vi "Read.vi"() -> ()   [LabVIEW 2017]
uses:
  <vilib>/Instr/_visa.llb/VISA Flush IO Buffer Mask.ctl
  <vilib>/Instr/_visa.llb/VISA Configure Serial Port (Instr).vi
panel:
  out "Waveform":i32(graph)
  out "read buffer":string
  in  "Start":bool
  in  "USB Port":refnum<visa-resource-name>
  in  "baud rate (115200)":u32=9600
  in  "parity (0:none)":enum16{"None", "Odd", "Even", "Mark", "Space"}(ring)
  in  "data bits (8)":u16=8 min=5 max=8 step=1
  in  "stop bits (10: 1 bit)":u16(ring)=10 items=["1.0"=10, "1.5"=15, "2.0"=20]
  in  "flow control (0:none)":u16(ring) items=["None", "XON/XOFF", "RTS/CTS", "XON/XOFF & RTS/CTS", "DTR/DSR", "XON/XOFF & DTR/DSR"]
  # "Designed By : Pouya Mansournia"
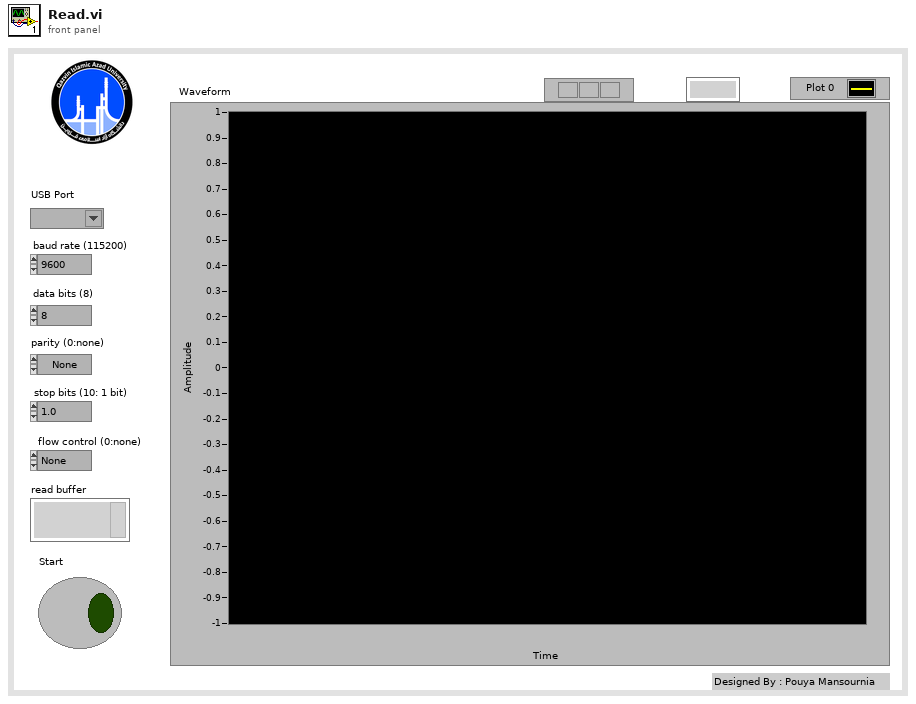
[diagram p1: front panel]
types:
  T1 = typedef "VISA Flush IO Buffer Mask.ctl" = u16
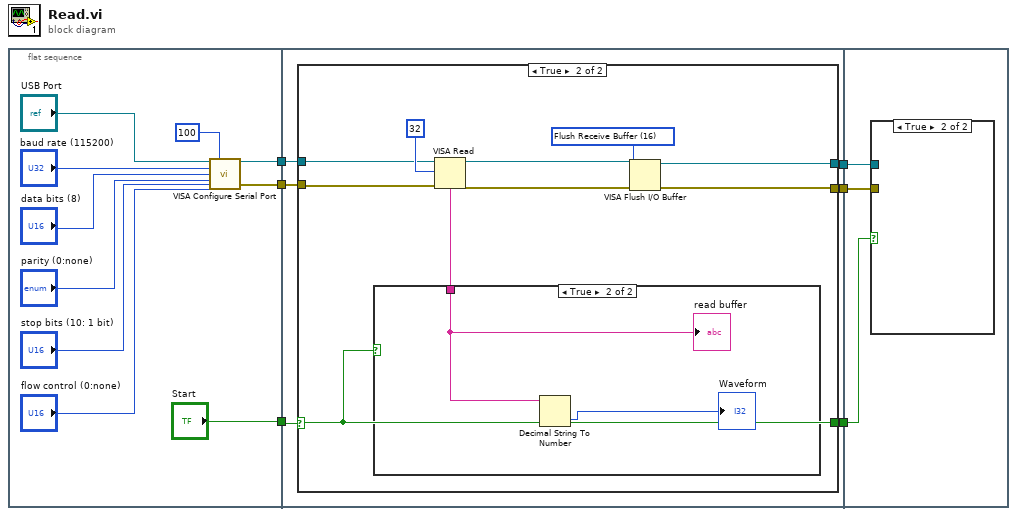
[diagram p0: block diagram]
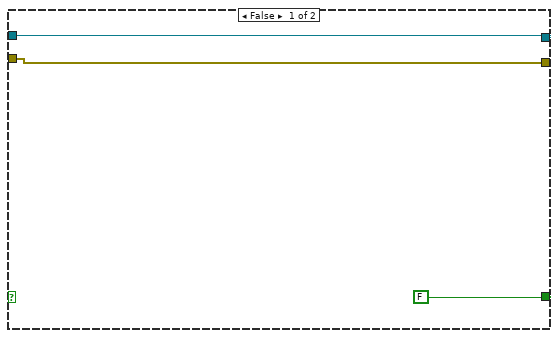
[diagram p2: hidden frame]
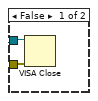
[diagram p4: hidden frame]
diagram:
  n1 = flat-sequence {
    tunnel: [w9] -> w6
    tunnel: [w10] -> w5
    tunnel: ["Start"] -> w2
    tunnel: w6 -> [w22]
    tunnel: w5 -> [w21]
    tunnel: [w20] -> w4
    tunnel: [w19] -> w3
    tunnel: w2 -> [w17]
    tunnel: [w18] -> w1
    tunnel: w4 -> [w40]
    tunnel: w3 -> [w39]
    tunnel: w1 -> [w38]
    frame #0 {
      n2 = call-poly "VISA Configure Serial Port"("VISA resource name"="USB Port", "timeout (10sec)"=u32 100, "baud rate (9600)"="baud rate (115200)", "data bits (8)"="data bits (8)", "parity (0:none)"="parity (0:none)", "stop bits (10: 1 bit)"="stop bits (10: 1 bit)", "flow control (0:none)"="flow control (0:none)") -> ("VISA resource name out"=w9:refnum<visa-resource-name>, "error out"=w10:errorcluster)  [unwired: 7 in]
    }
    frame #1 {
      n3 = case shown="True" w17 {
        selector: w17 -> [_ w29]
        tunnel: w22 -> [w25 w31]
        tunnel: w21 -> [w24 w26]
        tunnel: [w25 w30] -> w20
        tunnel: [w24 w28] -> w19
        tunnel: [FALSE w29] -> w18
        frame False {
        }
        frame True {
          w35 = T1 16 items=["Flush Receive Buffer"=16, "Write Transmit Buffer to Device"=32, "Flush Receive Buffer (No I/O)"=64, "Flush Transmit Buffer"=128] ("Mask")
          n4 = VISA Read(VISA resource name=w31, byte count=u32 32, error in (no error)=w26) -> (VISA resource name out=w34:refnum<visa-resource-name>, read buffer=w32:string, error out=w27:errorcluster)  [unwired: 1 out]
          n5 = case shown="True" w29 {
            tunnel: w32 -> [_ w37]
            frame False {
            }
            frame True {
              n6 = Decimal String To Number(string=w37) -> (number=→"Waveform":i32)  [unwired: 2 in, 1 out]
              "read buffer" <- w37
            }
          }
          n7 = VISA Flush I/O Buffer(VISA resource name=w34, mask (16)=w35, error in (no error)=w27) -> (VISA resource name out=w30:refnum<visa-resource-name>, error out=w28:errorcluster)
        }
      }
    }
    frame #2 {
      n8 = case shown="True" w38 {
        tunnel: w40 -> [w41 _]
        tunnel: w39 -> [w42 _]
        frame False {
          n9 = VISA Close(VISA resource name=w41, error in (no error)=w42) -> ()  [unwired: 1 out]
        }
        frame True {
        }
      }
    }
  }
